vi "String to Variant.vi"(10 "String":string, 11 "Type":variant) -> (2 "error out":errorcluster, 3 "Value":variant, 5 "Invalid Format":bool)   [LabVIEW 2020, in "FlexBlocks.lvlib"]
uses:
  FlexBlocks.lvlib
  <vilib>/Utility/Data Type/NI_Data Type.lvlib
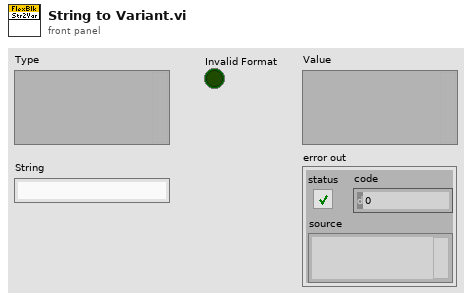
[diagram p1: front panel]
types:
  T1 = typedef "NI_Data Type.lvlib/Data Type.ctl" = enum8{"Invalid Type", "Void", "I8", "I16", "I32", "I64", "U8", "U16", "U32", "U64", "Single Float", "Double Float", "Extended Float", "Single Complex", "Double Complex", "Extended Complex", "Enum U8", "Enum U16", "Enum U32", "Enum U64", "Single Float With Unit", "Double Float With Unit", "Extended Float With Unit", "Single Complex with Unit", "Double Complex with Unit", "Extended Complex with Unit", "Boolean", "String", "Path", "Picture", "Tag", "Array", "Cluster", "Variant", "LV Variant", "Waveform", "Timestamp", "Digital Waveform", "Digital Data", "ExpressData", "Refnum", "External Data", "VI", "Poly VI", "LabVIEW Class Instance", "Fixed Point", "Set Collection", "Map Collection"}
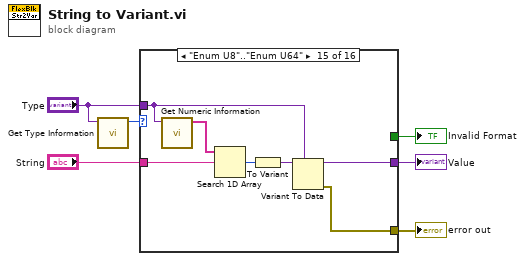
[diagram p0: block diagram]
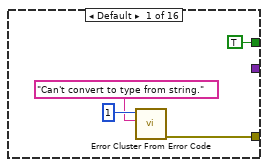
[diagram p2: hidden frame]
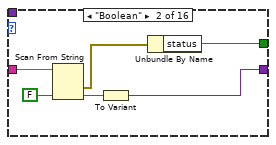
[diagram p3: hidden frame]
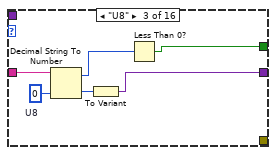
[diagram p4: hidden frame]
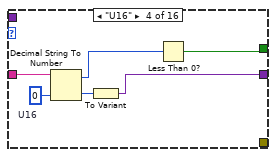
[diagram p5: hidden frame]
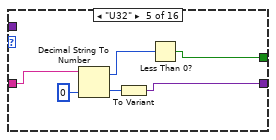
[diagram p6: hidden frame]
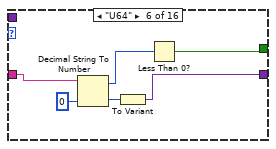
[diagram p7: hidden frame]
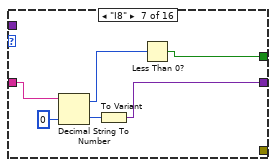
[diagram p8: hidden frame]
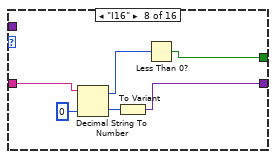
[diagram p9: hidden frame]
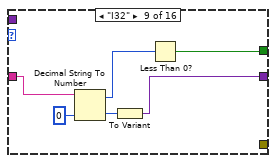
[diagram p10: hidden frame]
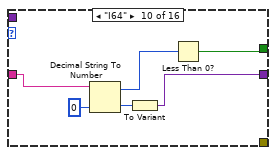
[diagram p11: hidden frame]
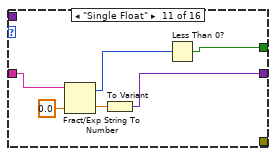
[diagram p12: hidden frame]
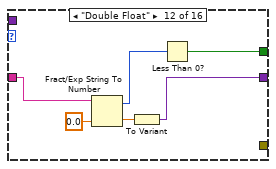
[diagram p13: hidden frame]
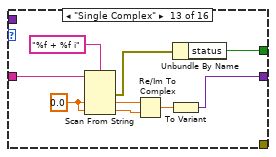
[diagram p14: hidden frame]
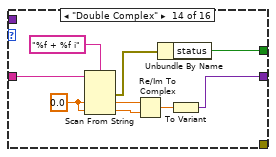
[diagram p15: hidden frame]
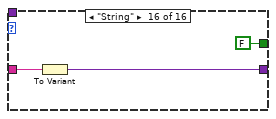
[diagram p16: hidden frame]
diagram:
  n1 = call <vilib>:"Get Type Information.vi"("variant"="Type") -> ("type"=w6:T1)  [unwired: 6 in, 4 out]
  n2 = case shown="\"Enum U8\"..\"Enum U64\"" w6 {
    tunnel: "String" -> [_ w16 w22 w26 w32 w38 w44 w50 w56 w62 w68 w74 w85 w94 w101 w104]
    tunnel: [_ w13 w19 w25 w31 w37 w43 w49 w55 w61 w67 w73 w79 w88 w96 w103] -> w4
    tunnel: [w8 _ _ _ _ _ _ _ _ _ _ _ _ _ w95 _] -> w2
    tunnel: [TRUE ("status") w11 w17 w23 w29 w35 w41 w47 w53 w59 w65 w71 w77 w86 _ FALSE ("status")] -> w3
    tunnel: "Type" -> [_ _ _ _ _ _ _ _ _ _ _ _ _ _ w97 _]
    frame Default {
      n3 = call <vilib>:"Error Cluster From Error Code.vi"("error message (\"\")"="Can't convert to type from string." ("error message (\"\")"), "error code (0)"=1) -> ("error out"=w8:errorcluster)  [unwired: 7 in]
    }
    frame "Boolean" {
      n4 = Scan From String(input string=w16, default 1=FALSE) -> (error out=w12:errorcluster, output 1=w14:bool)  [unwired: 3 in, 2 out]
      n5 = To Variant(anything=w14) -> (Variant=w13:variant)
      n6 = Unbundle By Name(w12) -> ("status"=w11:bool)
    }
    frame "U8" {
      w21 = u8 0  # U8
      n7 = Decimal String To Number(string=w22, default (0L)=w21) -> (offset past number=w18:i32, number=w20:u8)  [unwired: 1 in]
      n8 = To Variant(anything=w20) -> (Variant=w19:variant)
      n9 = Less Than 0?(x=w18) -> (x < 0?=w17:bool)
    }
    frame "U16" {
      w28 = u16 0  # U16
      n10 = Decimal String To Number(string=w26, default (0L)=w28) -> (offset past number=w24:i32, number=w27:u16)  [unwired: 1 in]
      n11 = To Variant(anything=w27) -> (Variant=w25:variant)
      n12 = Less Than 0?(x=w24) -> (x < 0?=w23:bool)
    }
    frame "U32" {
      n13 = Decimal String To Number(string=w32, default (0L)=u32 0 ("default (0 I32)")) -> (offset past number=w30:i32, number=w33:u32)  [unwired: 1 in]
      n14 = To Variant(anything=w33) -> (Variant=w31:variant)
      n15 = Less Than 0?(x=w30) -> (x < 0?=w29:bool)
    }
    frame "U64" {
      n16 = Decimal String To Number(string=w38, default (0L)=u64 0 ("default (0 I32)")) -> (offset past number=w36:i32, number=w39:u64)  [unwired: 1 in]
      n17 = To Variant(anything=w39) -> (Variant=w37:variant)
      n18 = Less Than 0?(x=w36) -> (x < 0?=w35:bool)
    }
    frame "I8" {
      n19 = Decimal String To Number(string=w44, default (0L)=i8 0 ("default (0 I32)")) -> (offset past number=w42:i32, number=w45:i8)  [unwired: 1 in]
      n20 = To Variant(anything=w45) -> (Variant=w43:variant)
      n21 = Less Than 0?(x=w42) -> (x < 0?=w41:bool)
    }
    frame "I16" {
      n22 = Decimal String To Number(string=w50, default (0L)=i16 0 ("default (0 I32)")) -> (offset past number=w48:i32, number=w51:i16)  [unwired: 1 in]
      n23 = To Variant(anything=w51) -> (Variant=w49:variant)
      n24 = Less Than 0?(x=w48) -> (x < 0?=w47:bool)
    }
    frame "I32" {
      n25 = Decimal String To Number(string=w56, default (0L)=0 ("default (0 I32)")) -> (offset past number=w54:i32, number=w57:i32)  [unwired: 1 in]
      n26 = To Variant(anything=w57) -> (Variant=w55:variant)
      n27 = Less Than 0?(x=w54) -> (x < 0?=w53:bool)
    }
    frame "I64" {
      n28 = Decimal String To Number(string=w62, default (0L)=i64 0 ("default (0 I32)")) -> (offset past number=w60:i32, number=w63:i64)  [unwired: 1 in]
      n29 = To Variant(anything=w63) -> (Variant=w61:variant)
      n30 = Less Than 0?(x=w60) -> (x < 0?=w59:bool)
    }
    frame "Single Float" {
      n31 = Fract/Exp String To Number(string=w68, default (0 dbl)=sgl 0.0 ("default (0 I32)")) -> (offset past number=w66:i32, number=w69:sgl)  [unwired: 2 in]
      n32 = To Variant(anything=w69) -> (Variant=w67:variant)
      n33 = Less Than 0?(x=w66) -> (x < 0?=w65:bool)
    }
    frame "Double Float" {
      n34 = Fract/Exp String To Number(string=w74, default (0 dbl)=sgl 0.0 ("default (0 I32)")) -> (offset past number=w72:i32, number=w75:sgl)  [unwired: 2 in]
      n35 = To Variant(anything=w75) -> (Variant=w73:variant)
      n36 = Less Than 0?(x=w72) -> (x < 0?=w71:bool)
    }
    frame "Single Complex" {
      w83 = sgl 0.0 ("default value 1")
      n37 = Scan From String(format string="%f + %f i", input string=w85, default 1=w83, default 2=w83) -> (error out=w78:errorcluster, output 1=w82:sgl, output 2=w81:sgl)  [unwired: 2 in, 2 out]
      n38 = Re/Im To Complex(1:w81, 2:w82) -> (0:w80:csg)
      n39 = To Variant(anything=w80) -> (Variant=w79:variant)
      n40 = Unbundle By Name(w78) -> ("status"=w77:bool)
    }
    frame "Double Complex" {
      w92 = 0.0 ("default value 1")
      n41 = Scan From String(format string="%f + %f i", input string=w94, default 1=w92, default 2=w92) -> (error out=w87:errorcluster, output 1=w91:dbl, output 2=w90:dbl)  [unwired: 2 in, 2 out]
      n42 = Re/Im To Complex(1:w90, 2:w91) -> (0:w89:cdb)
      n43 = Unbundle By Name(w87) -> ("status"=w86:bool)
      n44 = To Variant(anything=w89) -> (Variant=w88:variant)
    }
    frame "Enum U8".."Enum U64" {
      n45 = call <vilib>:"Get Numeric Information.vi"("variant"=w97) -> ("enum names"=w100:string[])  [unwired: 7 in, 3 out]
      n46 = Search 1D Array(1D array=w100, element=w101) -> (index of element=w99:i32)  [unwired: 1 in]
      n47 = To Variant(anything=w99) -> (Variant=w98:variant)
      n48 = Variant To Data(type=w97, Variant=w98) -> (data=w96:variant, error out=w95:errorcluster)  [unwired: 1 in]
    }
    frame "String" {
      n49 = To Variant(anything=w104) -> (Variant=w103:variant)
    }
  }
  "Value" <- w4
  "Invalid Format" <- w3
  "error out" <- w2
